vi "Impedance Echem.vi"(0 "Capacitance Functional Molecules per NS":dbl, 1 "C_EDL/ 1 NS":dbl, 5 "Series Resistance of Solution":dbl, 7 "Frequency":dbl, 9 "Freq Hz-MHz":dbl, 12 "Capacitance Functional Analyte per NS":dbl) -> (2 "Delta Total Impedance":dbl, 3 "Total Impedance Rs+C(EDS+Funct+Analyte)":dbl, 4 "Total Impedance Rs+C(EDS+Funct)":dbl, 6 "Impedance of EDL & Functionalization":dbl, 8 "Impedance of EDL & Functionalization & Analyte":dbl, 10 "Capacitance of ELD & Functionalization":dbl, 13 "Delta C":dbl, 14 "Capacitance of ELD & Functionalization & Analyte":dbl)   [LabVIEW 2020]
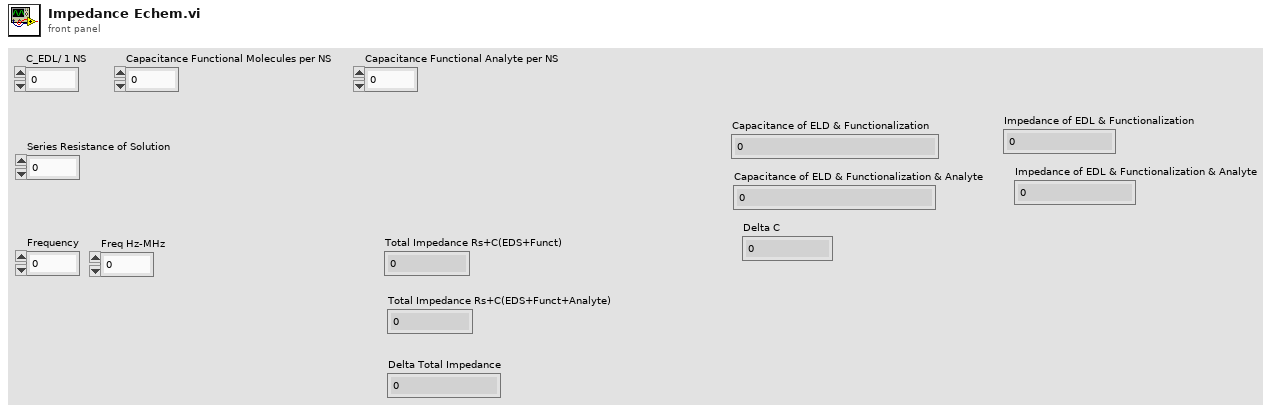
[diagram p1: front panel]
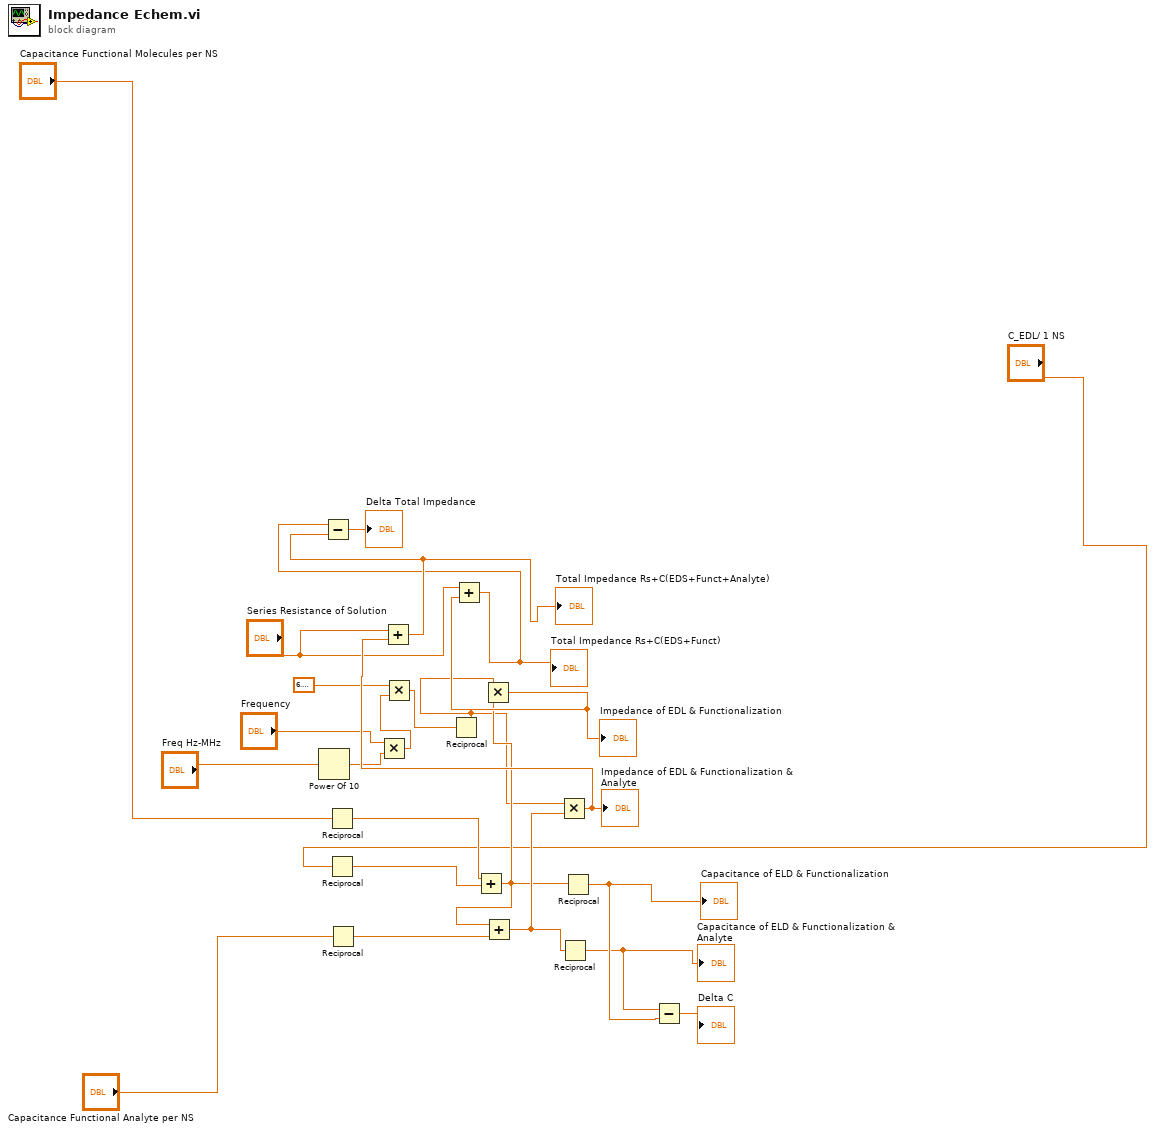
[diagram p0: block diagram]
diagram:
  n1 = Power Of 10(x="Freq Hz-MHz") -> (10^x=w17:dbl)
  n2 = Reciprocal(x="Capacitance Functional Molecules per NS") -> (1/x=w4:dbl)
  n3 = Reciprocal(x="C_EDL/ 1 NS") -> (1/x=w5:dbl)
  n4 = Reciprocal(x="Capacitance Functional Analyte per NS") -> (1/x=w6:dbl)
  n5 = Multiply(x="Frequency", y=w17) -> (x*y=w15:dbl)
  n6 = Multiply(x=6.283185307179586, y=w15) -> (x*y=w11:dbl)
  n7 = Reciprocal(x=w11) -> (1/x=w12:dbl)
  n8 = Add(x=w4, y=w5) -> (x+y=w13:dbl)
  n9 = Multiply(x=w12, y=w13) -> (x*y=w19:dbl)
  "Impedance of EDL & Functionalization" <- w19
  n10 = Add(x="Series Resistance of Solution", y=w19) -> (x+y=w23:dbl)
  "Total Impedance Rs+C(EDS+Funct)" <- w23
  n11 = Add(x=w13, y=w6) -> (x+y=w14:dbl)
  n12 = Multiply(x=w12, y=w14) -> (x*y=w21:dbl)
  "Impedance of EDL & Functionalization & Analyte" <- w21
  n13 = Add(x="Series Resistance of Solution", y=w21) -> (x+y=w24:dbl)
  "Total Impedance Rs+C(EDS+Funct+Analyte)" <- w24
  n14 = Subtract(x=w23, y=w24) -> (x-y=→"Delta Total Impedance":dbl)
  n15 = Reciprocal(x=w14) -> (1/x=w7:dbl)
  "Capacitance of ELD & Functionalization & Analyte" <- w7
  n16 = Reciprocal(x=w13) -> (1/x=w8:dbl)
  "Capacitance of ELD & Functionalization" <- w8
  n17 = Subtract(x=w7, y=w8) -> (x-y=→"Delta C":dbl)
